vi "irSensor.vi"() -> ()   [LabVIEW 2021]
uses:
  <vilib>/Instr/_visa.llb/VISA Configure Serial Port (Instr).vi
panel:
  out "IR Sensor2":bool
  out "IR Sensor1":bool
  out "DİKKAT":string
  in  "Serial Communication":refnum<visa-resource-name>
  in  "stop":bool
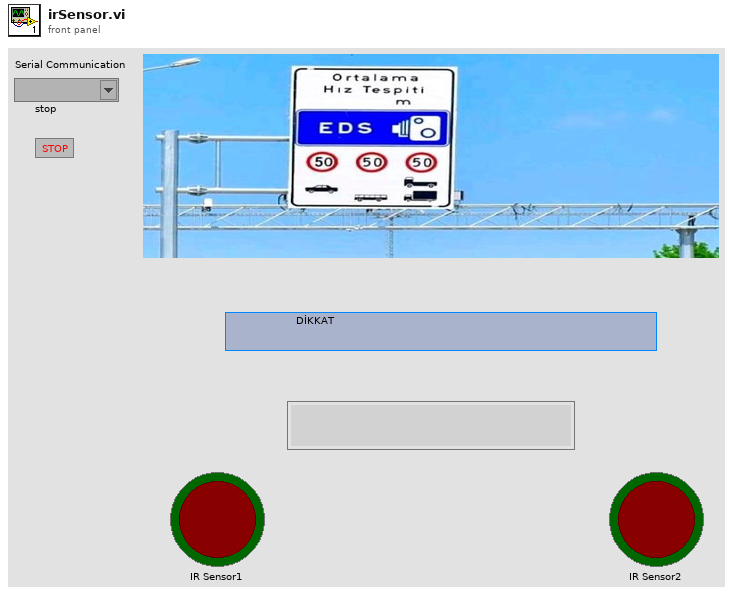
[diagram p1: front panel]
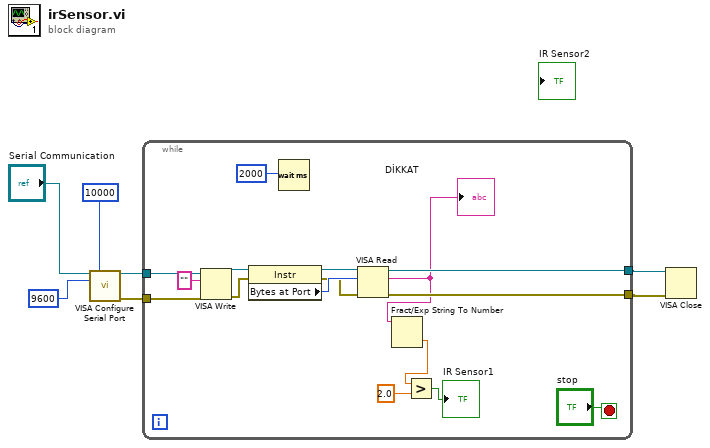
[diagram p0: block diagram]
diagram:
  n1 = call-poly "VISA Configure Serial Port"("VISA resource name"="Serial Communication", "timeout (10sec)"=u32 10000, "baud rate (9600)"=u32 9600) -> ("VISA resource name out"=w1:refnum<visa-resource-name>, "error out"=w2:errorcluster)  [unwired: 11 in]
  n2 = while {
    tunnel: [w22] -> w7
    tunnel: [w21] -> w6
    tunnel: w2 -> [w17]
    tunnel: w1 -> [w18]
    stop <- "stop" stop-if-true
    n3 = VISA Write(VISA resource name=w18, write buffer="", error in (no error)=w17) -> (VISA resource name out=w15:refnum<visa-resource-name>, error out=w16:errorcluster)  [unwired: 1 out]
    n4 = property class="Instr"(reference=w15, error in=w16) -> (reference out=w20:refnum<visa-resource-name>, error out=w12:errorcluster, "Bytes at Port"=w13:u32)
    n5 = Wait (ms)(milliseconds to wait=u32 2000) -> ()  [unwired: 1 out]
    n6 = VISA Read(VISA resource name=w20, byte count=w13, error in (no error)=w12) -> (VISA resource name out=w22:refnum<visa-resource-name>, read buffer=w11:string, error out=w21:errorcluster)  [unwired: 1 out]
    "DİKKAT" <- w11
    n7 = Fract/Exp String To Number(string=w11) -> (number=w10:dbl)  [unwired: 3 in, 1 out]
    n8 = Greater?(x=w10, y=2.0) -> (0:→"IR Sensor1":bool)
  }
  n9 = VISA Close(VISA resource name=w7, error in (no error)=w6) -> ()  [unwired: 1 out]
